vi "rs3 get api version.vi"(8 "error in (no error)":errorcluster) -> (0 "error out":errorcluster, 3 "version":i32=20000)   [LabVIEW 2023]
doc: "This retrieves the version number of the libRealSense library. \nThe output needs to be passed to Create Device."
panel:
  # "RS2 Get API Version"
  # "(C) Intel Corp.,  AGJ"
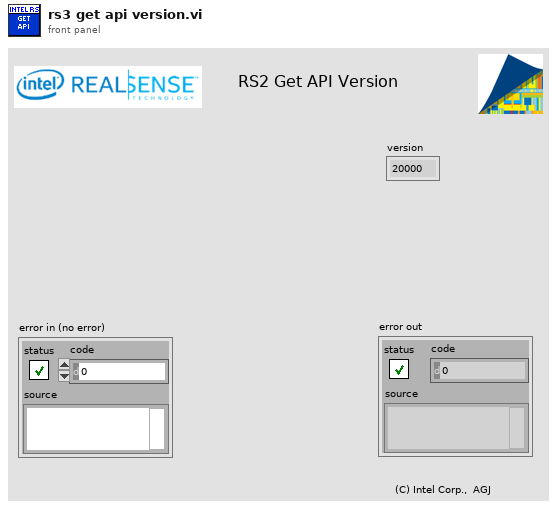
[diagram p1: front panel]
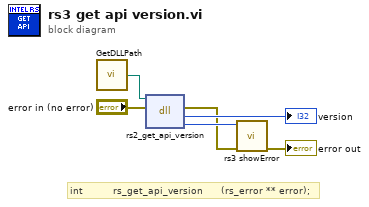
[diagram p0: block diagram]
diagram:
  # "int          rs_get_api_version      (rs_error ** error);"
  n1 = call "GetDLLPath.vi"() -> ("DLL Path"=w1:path)
  n2 = dll-call lib="C:/STEAMSyndicate/RealSenseWrappers/VI Wrappers (add ons) Public/RealSense/realsense2.dll" fn="rs2_get_api_version"(path in=w1, error in="error in (no error)") -> (error out=w3:errorcluster, "return type"=→"version":i32, "error"=w4:u64)  [unwired: 2 in, 1 out]
  n3 = call "rs3 showError.vi"("error in (no error)"=w3, "error"=w4) -> ("error out"=→"error out":errorcluster)  [unwired: 5 in, 4 out]
